vi "OCV_ACIR_Micro1.vi"(4 "R":dbl, 6 "V":dbl, 9 "V OK":bool, 10 "R OK":bool, 11 "DATA":T1) -> (3 "Tableau":string[](array[string]))   [LabVIEW 2020]
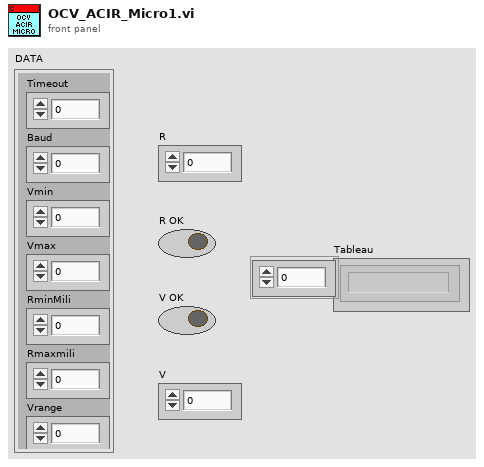
[diagram p1: front panel]
types:
  T1 = cluster{"Timeout":dbl, "Baud":u32, "Vmin":dbl, "Vmax":dbl, "RminMili":dbl, "Rmaxmili":dbl, "Vrange":dbl}
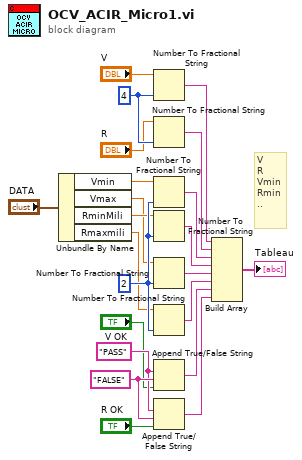
[diagram p0: block diagram]
diagram:
  w22 = i16 2 ("précision (6)")
  w6 = "FALSE"
  w5 = "PASS"
  w13 = i16 4 ("largeur (-)")
  # "V\nR\nVmin\nRmin\n.."
  n1 = Unbundle By Name("DATA") -> ("Vmin"=w18:dbl, "Vmax"=w19:dbl, "RminMili"=w20:dbl, "Rmaxmili"=w21:dbl)
  n2 = Number To Fractional String(number="V", precision (6)=w13) -> (F-format string=w10:string)  [unwired: 2 in]
  n3 = Number To Fractional String(number="R", precision (6)=w13) -> (F-format string=w11:string)  [unwired: 2 in]
  n4 = Number To Fractional String(number=w18, precision (6)=w22) -> (F-format string=w14:string)  [unwired: 2 in]
  n5 = Number To Fractional String(number=w20, precision (6)=w22) -> (F-format string=w15:string)  [unwired: 2 in]
  n6 = Number To Fractional String(number=w19, precision (6)=w22) -> (F-format string=w16:string)  [unwired: 2 in]
  n7 = Number To Fractional String(number=w21, precision (6)=w22) -> (F-format string=w17:string)  [unwired: 2 in]
  n8 = Append True/False String(1:"V OK", 2:w6, 3:w5) -> (0:w7:string)  [unwired: 1 in]
  n9 = Append True/False String(1:"R OK", 2:w6, 3:w5) -> (0:w8:string)  [unwired: 1 in]
  n10 = Build Array(w10, w11, w14, w15, w16, w17, w7, w8) -> (→"Tableau":string[])
